vi "Square wave.vi"(8 "Error In":errorcluster, 10 "Square wave settings":T1={"Square Chan"=0, "Low Value"=0.0, "High Value"=0.0, "Frequency"=1.0, "Duty Cycle"=50} {"Duty Cycle" min=1 max=99 step=1 format="%#_g %%"; "Frequency" min=0.5 max=500.0 step=0.5 format="%#_g Hz"; "High Value" min=0 max=204.8 step=0.0125 format="%#_g V"; "Low Value" min=0 max=204.8 step=0.0125 format="%#_g V"; "Square Chan" max=31 step=1}, 11 "Arduino Port":refnum<visa-resource-name>) -> (0 "Error Out":errorcluster, 3 "Arduino Port out":refnum<visa-resource-name>)   [LabVIEW 2016]
doc: "This VI execute a single period of square wave at Frequency between Low Value and High Value on the Channel"
uses:
  Typedef/AD5535 - Square wave settings.ctl
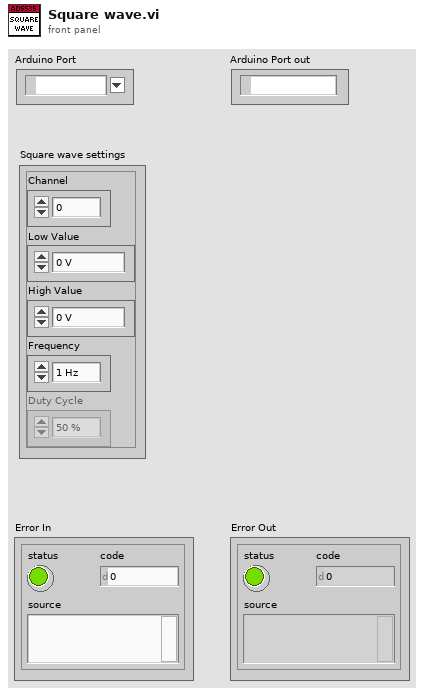
[diagram p1: front panel]
types:
  T1 = typedef "AD5535 - Square wave settings.ctl" = cluster{"Square Chan":u8, "Low Value":sgl, "High Value":sgl, "Frequency":dbl, "Duty Cycle":u8}
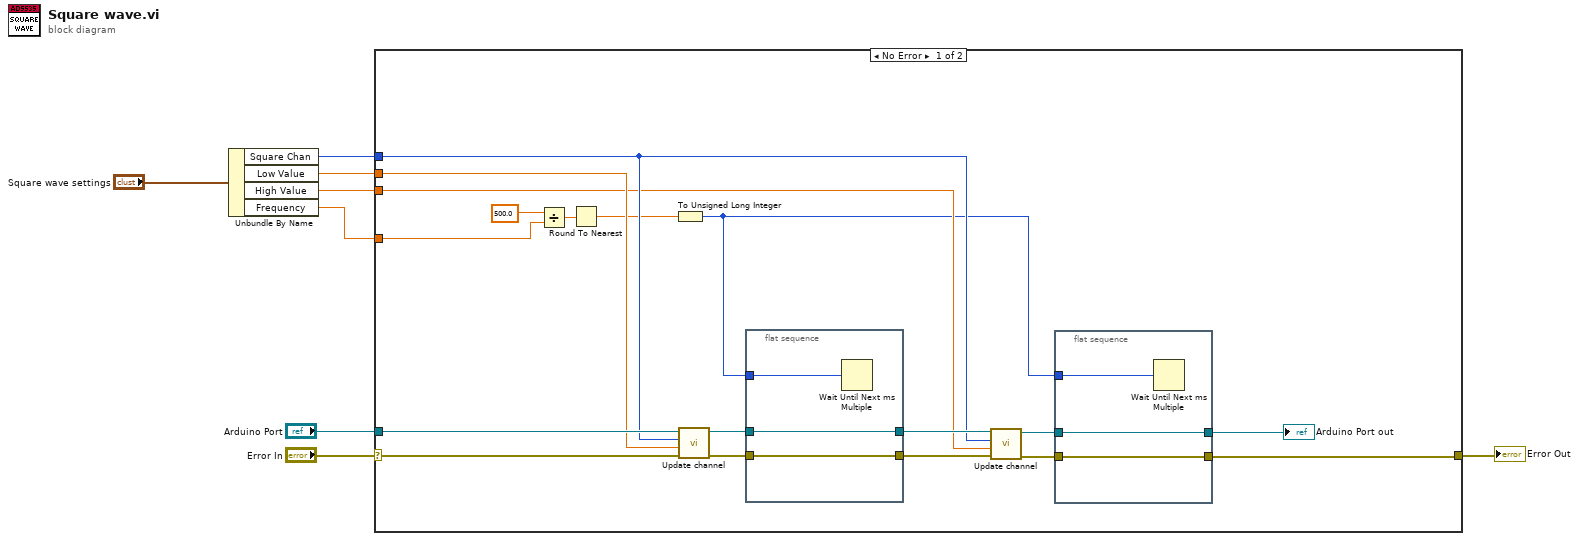
[diagram p0: block diagram]
diagram:
  n1 = Unbundle By Name("Square wave settings") -> ("Square Chan"=w4:u8, "Low Value"=w3:sgl, "High Value"=w2:sgl, "Frequency"=w1:dbl)
  n2 = case shown="No Error" "Error In" {
    selector: "Error In" -> [w26 w33]
    tunnel: [w18 w33] -> w7
    tunnel: "Arduino Port" -> [w25 _]
    tunnel: w4 -> [w16 _]
    tunnel: w3 -> [w15 _]
    tunnel: w2 -> [w14 _]
    tunnel: w1 -> [w9 _]
    frame No Error {
      n3 = Divide(x=500.0 ("y"), y=w9) -> (x/y=w13:dbl)
      n4 = Round To Nearest(number=w13) -> (nearest integer value=w12:dbl)
      n5 = To Unsigned Long Integer(number=w12) -> (unsigned 32bit integer=w11:u32)
      n6 = call "Update channel.vi"("Error In"=w26, "Value"=w15, "Channel"=w16, "Arduino Port"=w25) -> ("Error Out"=w23:errorcluster, "Arduino Port out"=w24:refnum<visa-resource-name>)  [unwired: 6 in]
      n7 = flat-sequence {
        tunnel: w24 -> [w32]
        tunnel: w23 -> [w31]
        tunnel: [w32] -> w20
        tunnel: [w31] -> w19
        tunnel: w11 -> [w30]
        frame #0 {
          n8 = Wait Until Next ms Multiple(millisecond multiple=w30) -> ()  [unwired: 1 out]
        }
      }
      n9 = call "Update channel.vi"("Error In"=w19, "Value"=w14, "Channel"=w16, "Arduino Port"=w20) -> ("Error Out"=w21:errorcluster, "Arduino Port out"=w22:refnum<visa-resource-name>)  [unwired: 6 in]
      n10 = flat-sequence {
        tunnel: w22 -> [w29]
        tunnel: w21 -> [w28]
        tunnel: [w29] -> w17
        tunnel: [w28] -> w18
        tunnel: w11 -> [w27]
        frame #0 {
          n11 = Wait Until Next ms Multiple(millisecond multiple=w27) -> ()  [unwired: 1 out]
        }
      }
      "Arduino Port out" <- w17
    }
    frame Error {
    }
  }
  "Error Out" <- w7
